vi "GetText.vi"(8 "error in":errorcluster, 11 "shared memory module editor node":refnum<class "Shared Memory Editor Node.lvclass">) -> (0 "error out":errorcluster, 1 "additional text":string, 2 "text":string, 3 "shared memory module editor node out":refnum<class "Shared Memory Editor Node.lvclass">, 4 "glyph":string)   [LabVIEW 2013, in "Shared Memory Editor Node.lvclass"]
doc: "Copyright 2016 National Instruments Corporation\n\nLicensed under the Apache License, Version 2.0 (the \"License\"); you may not use this file except in compliance with the License. You may obtain a copy of the License at http://www.apache.org/licenses/LICENSE-2.0\nUnless required by applicable law or agreed to in writing, software distributed under the License is distributed on an \"AS IS\" BASIS, WITHOUT WARRANTIES OR CONDITIONS OF ANY KIND, either express or implied. See the License for the specific language governing permissions and limitations under the License."
uses:
  Shared Memory Editor Node.lvclass
  Shared Memory Editor Node.lvclass/Shared Memory Editor Node.ctl
  <vilib>/NI/Configuration Framework/serializable configuration/get alias.vi
  module/configuration/Shared Memory Configuration.lvclass
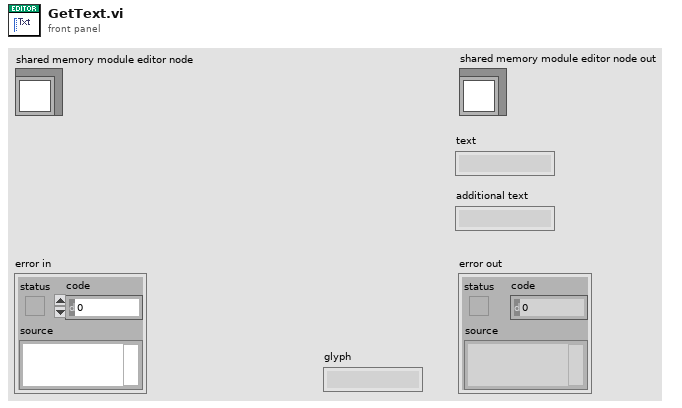
[diagram p1: front panel]
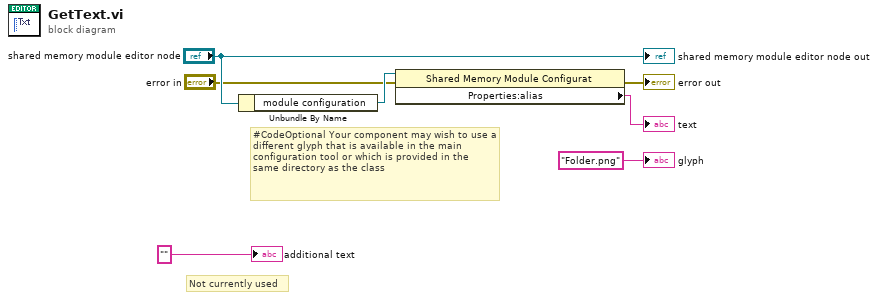
[diagram p0: block diagram]
diagram:
  # "Not currently used"
  # "#CodeOptional Your component may wish to use a different glyph that is available in the main configuration tool or which is provided in the same directory as the class"
  n1 = Unbundle By Name("shared memory module editor node") -> ("module configuration"=w4:refnum<class "Shared Memory Configuration.lvclass">)
  n2 = property class="Shared Memory Module Configurat"(reference=w4, error in="error in") -> (error out=→"error out":errorcluster, "Properties:alias"=→"text":string)  [unwired: 1 out]
  "shared memory module editor node out" <- "shared memory module editor node"
  "additional text" <- "" ("additional text")
  "glyph" <- "Folder.png" ("glyph")
